vi "start.vi"(8 "error in (no error)":errorcluster) -> (0 "error out":errorcluster)   [LabVIEW 2015, in "lv-launcher-nre.lvlib"]
uses:
  lv-launcher-nre.lvlib
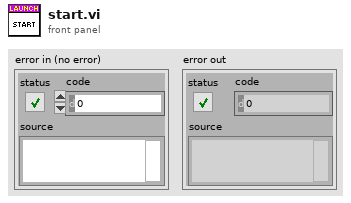
[diagram p1: front panel]
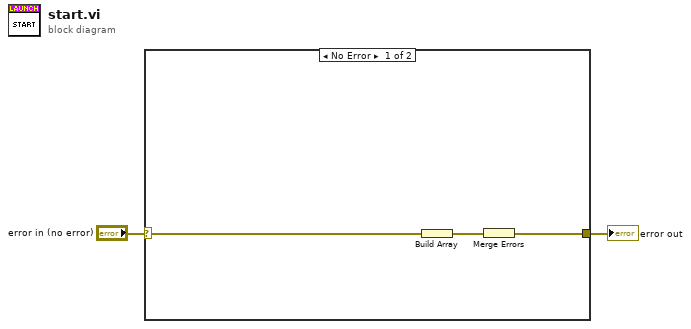
[diagram p0: block diagram]
diagram:
  n1 = case shown="No Error" "error in (no error)" {
    selector: "error in (no error)" -> [w4 w6]
    tunnel: [w5 w6] -> w1
    frame No Error {
      n2 = Build Array(w4) -> (w3:errorcluster[])
      n3 = Merge Errors(w3) -> (w5:errorcluster)
    }
    frame Error {
    }
  }
  "error out" <- w1
